vi "string_to_number.vi"(11 "String":string) -> (2 "default (0 dbl)":dbl, 3 "conversionOK":bool)   [LabVIEW 2015]
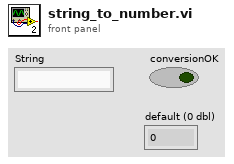
[diagram p1: front panel]
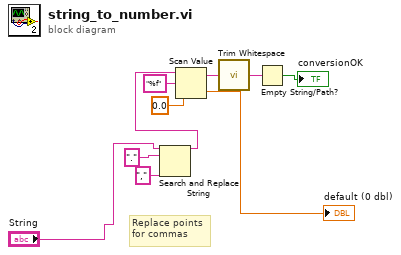
[diagram p0: block diagram]
diagram:
  # "Replace points\nfor commas"
  n1 = Search and Replace String(input string="String", search string=".", replace string="," ("replace string (\"\")")) -> (result string=w4:string)  [unwired: 5 in, 3 out]
  n2 = Scan Value(string=w4, format string="%f", default (0 dbl)=0.0) -> (output string=w1:string, value=→"default (0 dbl)":dbl)
  n3 = call <vilib>:"Trim Whitespace.vi"("string"=w1) -> ("trimmed string"=w2:string)  [unwired: 1 in]
  n4 = Empty String/Path?(string/path=w2) -> (empty?=→"conversionOK":bool)
